vi "demod_low.vi"(0 "Reset":bool, 5 "Config":T6={"IO params"={"Conversion"={"Rate"=4.0, "Num cards"=2, "Out channels"=4}, "Carriers"={"Phase shift"=180.0, "Levels"=[[0.8, 0.8, 0.8], [0.03, 0.03, 0.03]], "Delay samples"=73.15}, "TCP"={"Host"="192.168.1.15", "Port"=6666, "Buffering"=6, "Timeout"=6}, "Input channel sign"=[1, 1, 1]}, "High rate STFT"={"Win param"=101.5, "Window type"=61, "Win order"=2, "DFT size"=64, "Channels"=[7], "Oversample"=64}, "Low rate STFT"={"Win param"=120.0, "Window type"=61, "Win order"=8, "DFT size"=64, "Channels"=[7], "Oversample"=64}, "Filtering "=[]} {"Filtering"."Distortion"."Limit" format="%#_3p"; "Filtering"."Distortion"."LF cut" format="%#_3p"; "Filtering"."Kalman"."Measure noise" format="%#_3p"; "Filtering"."Kalman"."Process noise" format="%#_3p"; "Filtering"."Hum"."Limit" format="%#_3p"; "Filtering"."Hum"."Frequency" format="%#_4p"; "Low rate STFT"."Oversample" min=1 step=1; "Low rate STFT"."Channels" min=0 step=1; "Low rate STFT"."DFT size" min=1 step=1; "Low rate STFT"."Window type" items=["Rectangle"=0, "Hanning"=1, "Hamming"=2, "Blackman-Harris"=3, "Exact Blackman"=4, "Blackman"=5, "Flat Top"=6, "4 Term B-Harris "=7, "7 Term B-Harris"=8, "Low Sidelobe"=9, "Blackman Nuttall"=11, "Triangle"=30, "Bartlett-Hanning"=31, "Bohman"=32, "Parzen"=33, "Welch"=34, "Kaiser"=60, "Dolph-Chebyshev"=61, "Gaussian"=62]; "High rate STFT"."Oversample" min=1 step=1; "High rate STFT"."Channels" min=0 step=1; "High rate STFT"."DFT size" min=1 step=1; "High rate STFT"."Window type" items=["Rectangle"=0, "Hanning"=1, "Hamming"=2, "Blackman-Harris"=3, "Exact Blackman"=4, "Blackman"=5, "Flat Top"=6, "4 Term B-Harris "=7, "7 Term B-Harris"=8, "Low Sidelobe"=9, "Blackman Nuttall"=11, "Triangle"=30, "Bartlett-Hanning"=31, "Bohman"=32, "Parzen"=33, "Welch"=34, "Kaiser"=60, "Dolph-Chebyshev"=61, "Gaussian"=62]; "IO params"."Input channel sign" min=-1 max=1 step=1; "IO params"."Carriers"."Levels" min=0.0 step=0.1; "IO params"."Conversion"."Rate" format="%#_8g"}, 7 "Modulation info":T2={"Fs full"=0.0, "Fs high"=0.0, "Fs low"=0.0, "Read size"=0, "FFT size low"=5000, "df low"=5000.0, "High carriers"=[], "Low carriers"=[], "Hi channels at low"=[7]} {"Hi channels at low" min=0 step=1; "Low carriers" format="%#_6p"; "High carriers" format="%#_6p"}, 9 "Input card":i32=1, 11 "Trace info in":T3, 12 "Raw data":dbl[][][](array[numeric])) -> (4 "Carrier amplitudes":T1 format="%#_3p", 15 "Trace info out":T3)   [LabVIEW 2026]
uses:
  ilemt_config.ctl
  system/IO_params.ctl
  stft_params.ctl
  <vilib>/Analysis/4window.llb/windowTd.ctl
  filter_params.ctl
  detrend_mode.ctl
  gui/trace_info.ctl
  gui/trace_channel.ctl
  main/ilemt_status.ctl
  modulation_info.ctl
  carrier_amplitudes.ctl
  <vilib>/Analysis/NI_AALPro.lvlib
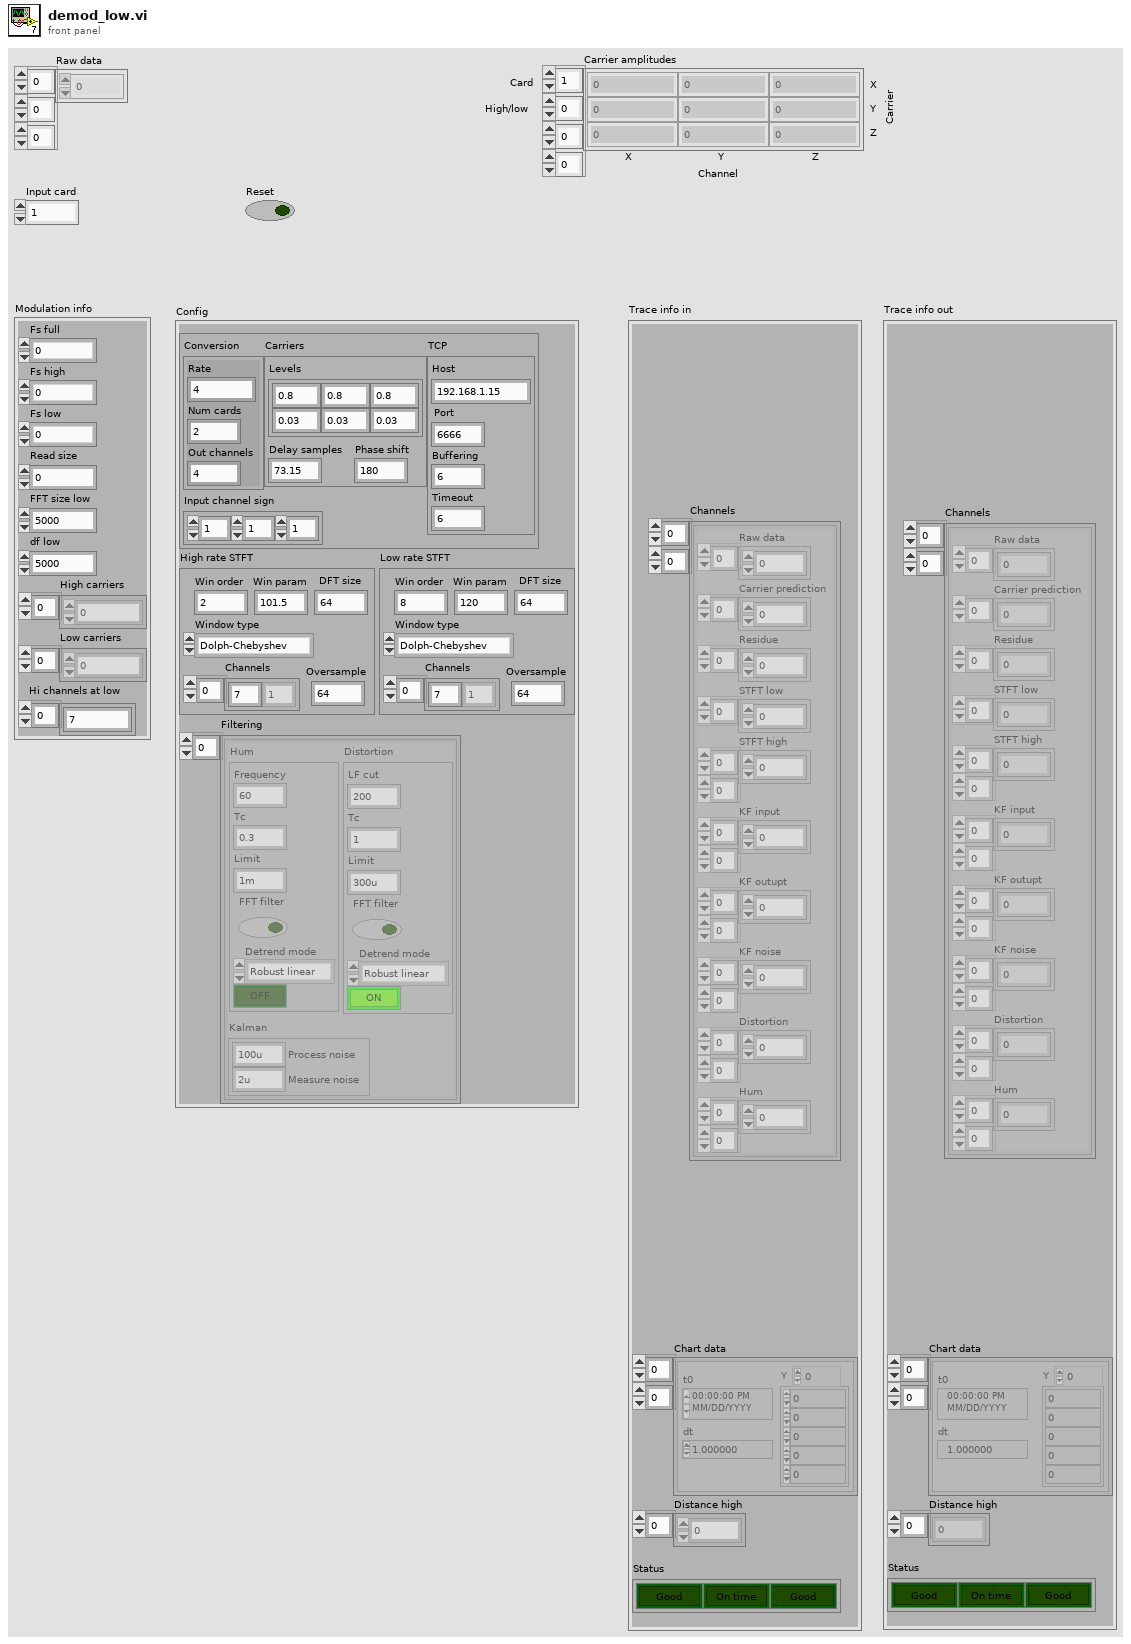
[diagram p1: front panel]
types:
  T1 = typedef "carrier_amplitudes.ctl" = cdb[][][][]
  T2 = typedef "modulation_info.ctl" = cluster{"Fs full":dbl, "Fs high":dbl, "Fs low":dbl, "Read size":i32, "FFT size low":i32, "df low":dbl, "High carriers":dbl[], "Low carriers":dbl[], "Hi channels at low":i32[]}
  T3 = typedef "trace_info.ctl" = cluster{"Channels":T4[][], "Chart data":waveform(dbl)[][], "Distance high":dbl[], "Status":T5}
  T4 = typedef "trace_channel.ctl" = cluster{"Raw data":dbl[], "Carrier prediction":dbl[], "Residue":dbl[], "STFT low":cdb[], "STFT high":cdb[][], "KF input":cdb[][], "KF outupt":cdb[][], "KF noise":dbl[][], "Distortion":cdb[][], "Hum":cdb[][]}
  T5 = typedef "ilemt_status.ctl" = cluster{"NaN":bool, "Backlog":bool, "Clipping":bool}
  T6 = typedef "ilemt_config.ctl" = cluster{"IO params":T7, "High rate STFT":T8, "Low rate STFT":T8, "Filtering ":T10[]}
  T7 = typedef "IO_params.ctl" = cluster{"Conversion":cluster{"Rate":dbl, "Num cards":u32, "Out channels":u32}, "Carriers":cluster{"Phase shift":dbl, "Levels":dbl[][], "Delay samples":dbl}, "TCP":cluster{"Host":string, "Port":i32, "Buffering":u32, "Timeout":u32}, "Input channel sign":i32[]}
  T8 = typedef "stft_params.ctl" = cluster{"Win param":dbl, "Window type":T9, "Win order":i32, "DFT size":i32, "Channels":i32[], "Oversample":i32}
  T9 = typedef "NI_AALPro.lvlib/windowTd.ctl" = u32
  T10 = typedef "filter_params.ctl" = cluster{"Hum":cluster{"Frequency":dbl, "Tc":dbl, "Limit":dbl, "FFT filter":bool, "Detrend mode":T11, "Enable":bool}, "Kalman":cluster{"Process noise":dbl, "Measure noise":dbl}, "Distortion":cluster{"LF cut":dbl, "Tc":dbl, "Limit":dbl, "FFT filter":bool, "Detrend mode":T11, "Enable":bool}}
  T11 = typedef "detrend_mode.ctl" = enum16{"Zero mean", "Linear", "Robust linear"}
  T12 = typedef "card_carrier_amplitudes.ctl" = cdb[][][]
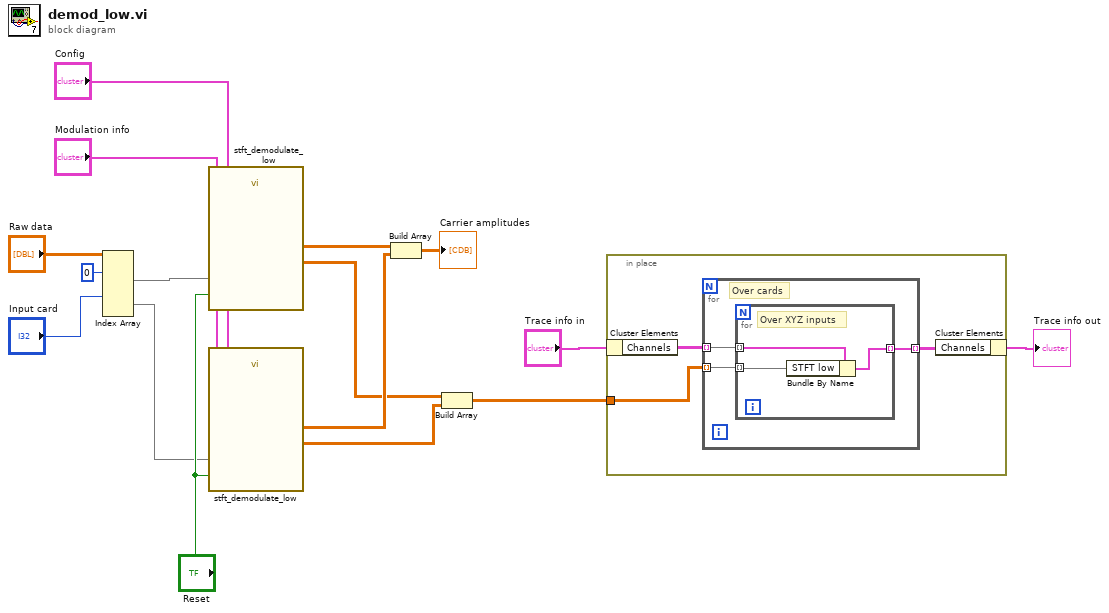
[diagram p0: block diagram]
diagram:
  n1 = Index Array(array="Raw data", index (dim 0) #1=0 ("index (page)"), index (dim 0) #2="Input card") -> (element #1=w11:dbl[][], element #2=w7:dbl[][])  [unwired: 4 in]
  n2 = call "stft_demodulate_low.vi"("Reset"="Reset", "Config"="Config", "Modulation info"="Modulation info", "Raw data"=w11) -> ("STFT"=w3:cdb[][], "Card carrier amplitudes"=w6:T12)  [unwired: 6 in]
  n3 = call "stft_demodulate_low.vi"("Reset"="Reset", "Config"="Config", "Modulation info"="Modulation info", "Raw data"=w7) -> ("STFT"=w4:cdb[][], "Card carrier amplitudes"=w5:T12)  [unwired: 6 in]
  n4 = Build Array(w6, w5) -> (→"Carrier amplitudes":cdb[][][][])
  n5 = Build Array(w3, w4) -> (w2:cdb[][][])
  n6 = in-place {
    in-place-border: w2 -> [w18]
    n7 = in-place-cluster #1("Trace info in") -> ("Channels"=w19:T4[][])
    n8 = for {
      tunnel: w19 -> [w22] mode=indexing
      tunnel: w18 -> [w21] mode=indexing
      tunnel: [w20] -> w17 mode=indexing
      # "Over cards"
      n9 = for {
        tunnel: [w25] -> w20 mode=indexing
        tunnel: w22 -> [w24] mode=indexing
        tunnel: w21 -> [w23] mode=indexing
        # "Over XYZ inputs"
        n10 = Bundle By Name(cluster=w24, "STFT low"=w23) -> (w25:T4)
      }
    }
    n11 = in-place-cluster #1("Channels"=w17) -> (→"Trace info out":T3)
  }
